vi "Update In World.vi"(11 "Ship in":refnum<class "Ship.lvclass">) -> (3 "Ship out":refnum<class "Ship.lvclass">)   [LabVIEW 2015, in "Ship.lvclass"]
uses:
  Ship.lvclass
  Element/Element.lvclass
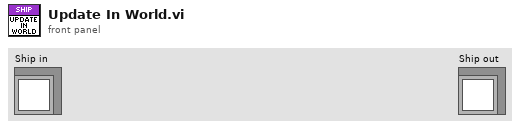
[diagram p1: front panel]
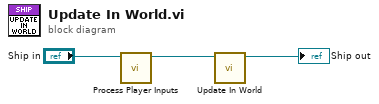
[diagram p0: block diagram]
diagram:
  n1 = call "Process Player Inputs.vi"("Ship in"="Ship in") -> ("Ship out"=w2:refnum<class "Ship.lvclass">)  [unwired: 10 in]
  n2 = call-parent "Update In World.vi"("Movable in"=w2) -> ("Movable out"=→"Ship out":refnum<class "Ship.lvclass">)  [unwired: 10 in]
